vi "FindValidBuildSpecs.vi"(8 "error in (no error)":errorcluster, 9 "Target Name":string, 10 "ProjectItem Refnums":refnum<vi>[](array[refnum]), 11 "ExecuteBuildSpecAllTargets in":refnum<class "ExecuteBuildSpecAllTargets.lvclass">) -> (0 "error out":errorcluster, 1 "Specs":T1[](array[typedef]), 2 "dup ProjectItem Refnums":refnum<vi>[](array[refnum]), 3 "ExecuteBuildSpecAllTargets out":refnum<class "ExecuteBuildSpecAllTargets.lvclass">)   [LabVIEW 2014, in "ExecuteBuildSpecAllTargets.lvclass"]
uses:
  ExecuteBuildSpecAllTargets.lvclass
  ExecuteMultipleBuildSpecs/SpecInformation.ctl
  ExecuteBuildSpecAllTargets.lvclass/ExecuteBuildSpecAllTargets.ctl
  ExecuteMultipleBuildSpecs/ExecuteMultipleBuildSpecs.lvclass
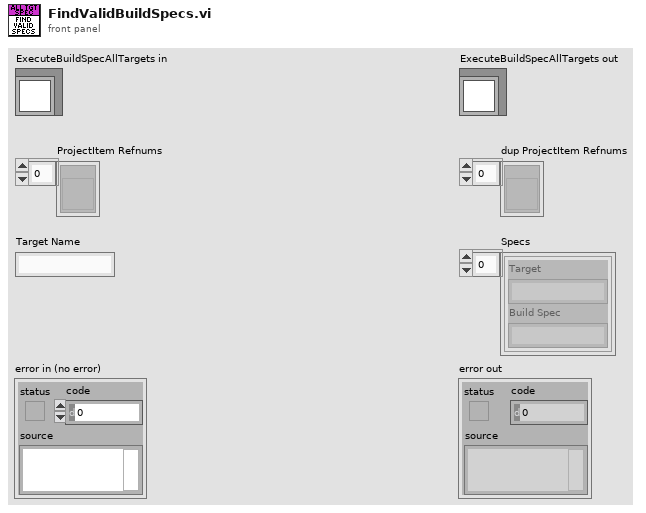
[diagram p1: front panel]
types:
  T1 = typedef "ExecuteMultipleBuildSpecs.lvclass/SpecInformation.ctl" = cluster{"Target":string, "Build Spec":string}
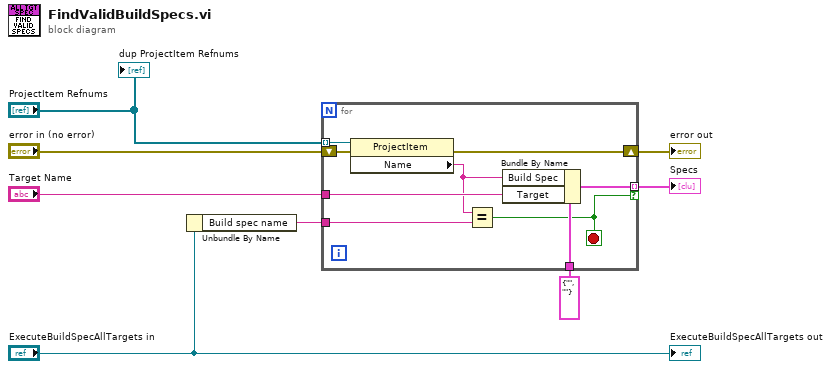
[diagram p0: block diagram]
diagram:
  n1 = Unbundle By Name("ExecuteBuildSpecAllTargets in") -> ("Build spec name"=w5:string)
  n2 = for {
    tunnel: "ProjectItem Refnums" -> [w16] mode=indexing
    shift-right: [w15] -> w4
    shift-left: "error in (no error)" -> [w17]
    tunnel: "Target Name" -> [w13]
    tunnel: T1 {"Target"="", "Build Spec"=""} ("Spec Info") -> [w14]
    tunnel: [w12] -> w3 mode=indexing if=w9
    tunnel: w5 -> [w10]
    stop <- w9 stop-if-true
    n3 = property class="ProjectItem"(reference=w16, error in=w17) -> (error out=w15:errorcluster, "Name"=w11:string)  [unwired: 1 out]
    n4 = Equal?(x=w11, y=w10) -> (x = y?=w9:bool)
    n5 = Bundle By Name(cluster=w14, "Build Spec"=w11, "Target"=w13) -> (w12:T1)
  }
  "error out" <- w4
  "Specs" <- w3
  "ExecuteBuildSpecAllTargets out" <- "ExecuteBuildSpecAllTargets in"
  "dup ProjectItem Refnums" <- "ProjectItem Refnums"
